vi "IV to IdVdI.vi"(10 "Array in":dbl[][](array[numeric])) -> (2 "Array":dbl[][](array[numeric]), 3 "Array 2":dbl[][](array[numeric]))   [LabVIEW 2024]
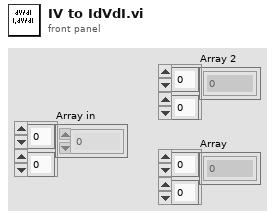
[diagram p1: front panel]
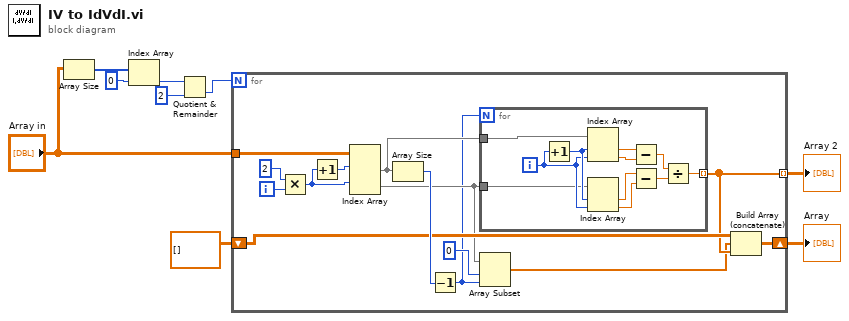
[diagram p0: block diagram]
diagram:
  n1 = Array Size(array="Array in") -> (size(s)=w5:i32[])
  n2 = Index Array(array=w5, index=0) -> (element=w3:i32)
  n3 = Quotient & Remainder(x=w3, y=2) -> (floor(x/y)=w1:i32)  [unwired: 1 out]
  n4 = for {
    N: w1 -> [_]
    tunnel: "Array in" -> [w23]
    tunnel: [w15] -> w7 mode=indexing
    shift-right: [w10] -> w9
    shift-left: dbl[][] [] -> [w16]
    i -> [w22]
    n5 = Multiply(x=2, y=w22) -> (x*y=w18:i32)
    n6 = Increment(x=w18) -> (x+1=w20:i32)
    n7 = Index Array(array=w23, index (row) #1=w20, index (row) #2=w18) -> (element #1=w17:dbl[], element #2=w14:dbl[])  [unwired: 2 in]
    n8 = Array Size(array=w17) -> (size(s)=w19:i32)
    n9 = Decrement(x=w19) -> (x-1=w12:i32)
    n10 = for {
      N: w12 -> [_]
      tunnel: w17 -> [w34]
      tunnel: w14 -> [w27]
      tunnel: [w24] -> w15 mode=indexing
      i -> [w28]
      n11 = Increment(x=w28) -> (x+1=w29:i32)
      n12 = Index Array(array=w34, index #1=w29, index #2=w28) -> (element #1=w33:dbl, element #2=w32:dbl)
      n13 = Index Array(array=w27, index #1=w29, index #2=w28) -> (element #1=w31:dbl, element #2=w30:dbl)
      n14 = Subtract(x=w33, y=w32) -> (x-y=w25:dbl)
      n15 = Subtract(x=w31, y=w30) -> (x-y=w26:dbl)
      n16 = Divide(x=w25, y=w26) -> (x/y=w24:dbl)
    }
    n17 = Array Subset(array=w14, index=0, length=w12) -> (w11:dbl[])
    n18 = Build Array (concatenate)(w16, w11, w15) -> (w10:dbl[][])
  }
  "Array" <- w9
  "Array 2" <- w7
